vi "Menu_unCheck.vi"(7 "Ctrl":string, 8 "error in (no error)":errorcluster, 10 "DB Ref":T1, 11 "String":string) -> (0 "error out":errorcluster)   [LabVIEW 2017, in "tagdb-RefMgr Operations.lvlib"]
uses:
  tagdb-RefMgr Operations.lvlib
  <userlib>/_NEVSTOP/TagDB/Typedef/TagDB.ctl
  00d0da00-135c-4b50-b029-f1f1f0d03544.vi
  3fef5895-5f1b-4d45-a284-c279625095f7.vi
  4c542a80-f847-4821-836c-1c9f0a826a9d.vi
  00d0da00-135c-4b50-b029-f1f1f0d03544.vi/1b47866c-8e2d-43a7-815f-8cf18635e5a1.vi
  4c542a80-f847-4821-836c-1c9f0a826a9d.vi/1b47866c-8e2d-43a7-815f-8cf18635e5a1.vi
  <userlib>/_NEVSTOP/TagDB/_Support/Error/_Clear Errors.vi
  00d0da00-135c-4b50-b029-f1f1f0d03544.vi/1b47866c-8e2d-43a7-815f-8cf18635e5a1.vi/29b2ea6d-6d7f-4e4a-ad31-a5cb760462c7.vi
  <userlib>/_NEVSTOP/TagDB/API/TagDB-Status.vi
  4c542a80-f847-4821-836c-1c9f0a826a9d.vi/1b47866c-8e2d-43a7-815f-8cf18635e5a1.vi/29b2ea6d-6d7f-4e4a-ad31-a5cb760462c7.vi
  <userlib>/_NEVSTOP/TagDB/_Support/DataAccess/_NameCacher.vi
  <userlib>/_NEVSTOP/TagDB/_Support/Change Detector/TagDB dbChanged.vi
  <userlib>/_NEVSTOP/TagDB/_Support/DataAccess/TagDB Ref to DVR.vi
  <userlib>/_NEVSTOP/TagDB/_Support/Error/_[error50000]Invalid DB REF.vi
  <userlib>/_NEVSTOP/TagDB/_Support/URL/TRIM-BOTH-SPACE.vi
  <userlib>/_NEVSTOP/TagDB/_Support/Error/_[error50002]Invalid DataType.vi
  <userlib>/_NEVSTOP/TagDB/TagDB.lvlib
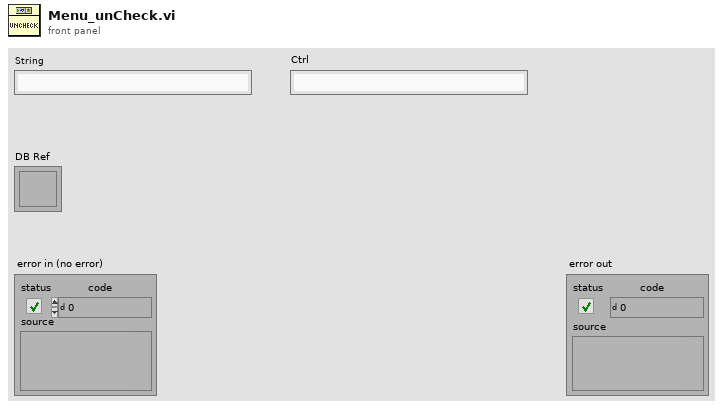
[diagram p1: front panel]
types:
  T1 = typedef "TagDB.lvlib/TagDB.ctl" = refnum<k1>
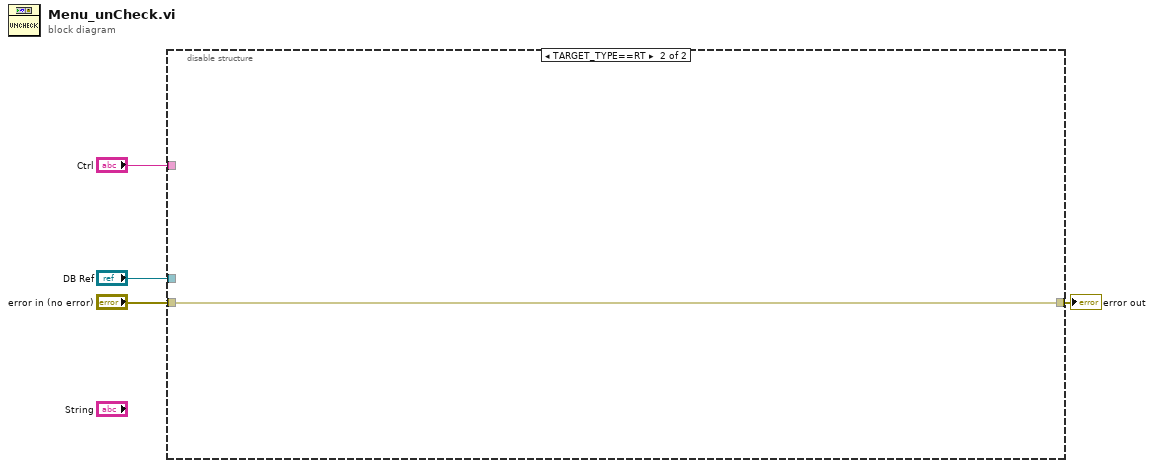
[diagram p0: block diagram]
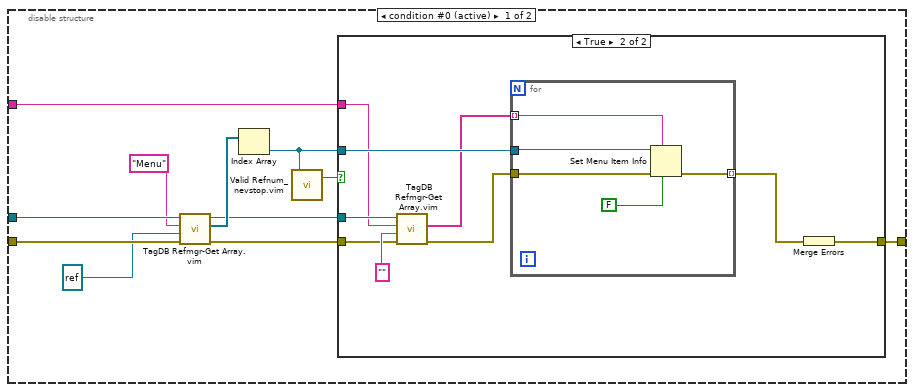
[diagram p2: hidden frame]
diagram:
  n1 = disable-structure shown="TARGET_TYPE==RT" {
    disable-tunnel: "error in (no error)" -> [w15 w31]
    disable-tunnel: "DB Ref" -> [w14 _]
    disable-tunnel: "Ctrl" -> [w8 _]
    disable-tunnel: [w7 w31] -> w1
    frame condition #0 (active) {
      n2 = call "TagDB Refmgr-Get Array.vim"("error in (no error)"=w15, "Type"=refnum<k9> refnum ("menu reference"), "RegExp"="Menu", "DB Ref"=w14) -> ("error out"=w6:errorcluster, "References"=w11:refnum<k9>[], "DB Ref(dup)"=w10:T1)  [unwired: 4 in, 1 out]
      n3 = Index Array(array=w11) -> (element=w9:refnum<k9>)  [unwired: 1 in]
      n4 = call "Valid Refnum_nevstop.vim"("number/path/refnum"=w9) -> ("Valid Number/Path/Refnum"=w5:bool)  [unwired: 2 in]
      n5 = case shown="True" w5 {
        tunnel: w10 -> [_ w25]
        tunnel: w9 -> [_ w24]
        tunnel: w8 -> [_ w22]
        tunnel: [w16 w19] -> w7
        tunnel: w6 -> [w16 w18]
        frame False {
        }
        frame True {
          n6 = call "TagDB Refmgr-Get Array.vim"("error in (no error)"=w18, "Type"="" ("RegExp"), "RegExp"=w22, "DB Ref"=w25) -> ("error out"=w17:errorcluster, "References"=w21:string[])  [unwired: 4 in, 2 out]
          n7 = for {
            tunnel: w24 -> [w30]
            tunnel: w21 -> [w28] mode=indexing
            tunnel: w17 -> [w27]
            tunnel: [w26] -> w20 mode=indexing
            n8 = Set Menu Item Info(6:FALSE ("checked"), 7:w28, 8:w27, 11:w30) -> (0:w26:errorcluster)  [unwired: 3 in, 1 out]
          }
          n9 = Merge Errors(w20) -> (w19:errorcluster)
        }
      }
    }
    frame condition #1 {
    }
  }
  "error out" <- w1
